vi "GetWyPts_Poloymorphic.vi"   [LabVIEW 2020, in "WyPtDict.lvlib"]
doc: "Developed by Kevin Thompson\nkevin@thompsonengineering.net\n\nCopyright 2021\nThompson Engineering, LLC"
uses:
  WyPtDict.lvlib
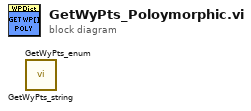
[diagram p0: block diagram]
diagram:
  n1 = call "GetWyPts_string.vi"() -> ()  [unwired: 7 in, 5 out]
  n2 = call "GetWyPts_enum.vi"() -> ()  [unwired: 7 in, 5 out]
